vi "X_Overlay Dashed Line.vi"(4 "Dash Length (0)":u32, 6 "Color":u32, 7 "Overlay Group":string, 8 "error in (no error)":errorcluster, 9 "Point 2":T2, 10 "Point 1":T2, 11 "Refnum in":T1) -> (0 "error out":errorcluster, 3 "Refnum out":T1)   [LabVIEW 2021, in "Image.lvlib"]
uses:
  <vilib>/vision/Image Controls.llb/IMAQ Image.ctl
  Image.lvlib
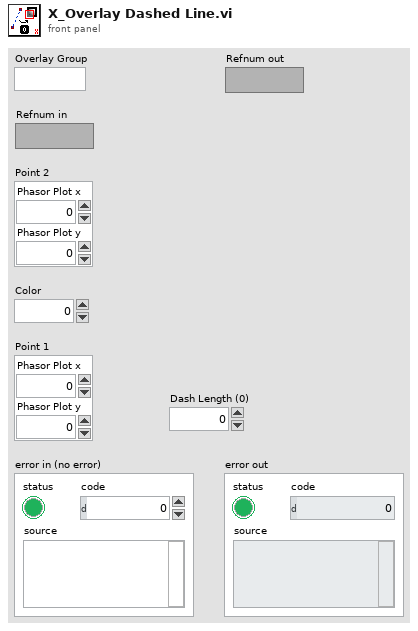
[diagram p1: front panel]
types:
  T1 = typedef "IMAQ Image.ctl" = refnum<image>
  T2 = cluster{"Phasor Plot x":i32, "Phasor Plot y":i32}
  T3 = cluster{"Phasor Plot x":i32, "Phasor Plot y":i32}[]
  T4 = cluster{"Phasor Plot x":dbl, "Phasor Plot y":dbl}
  T5 = cluster{"Phasor Plot x":dbl, "Phasor Plot y":dbl}[]
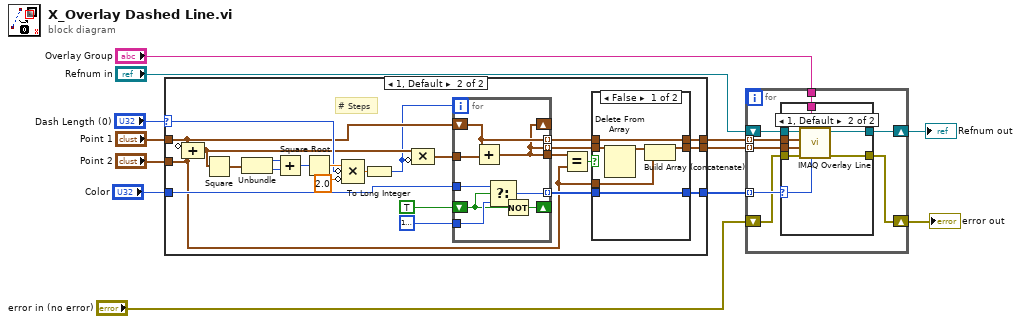
[diagram p0: block diagram]
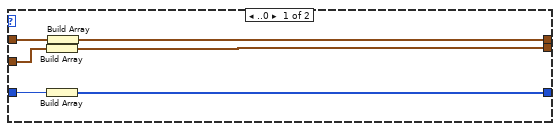
[diagram p2: hidden frame]
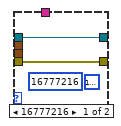
[diagram p4: hidden frame]
diagram:
  n1 = case shown="1, Default" "Dash Length (0)" {
    selector: "Dash Length (0)" -> [_ w37]
    tunnel: "Point 1" -> [w18 w35]
    tunnel: "Point 2" -> [w16 w19]
    tunnel: [w17 w23] -> w4
    tunnel: [w15 w22] -> w3
    tunnel: "Color" -> [w14 w33]
    tunnel: [w13 w20] -> w1
    frame ..0 {
      n2 = Build Array(w16) -> (w15:T3)
      n3 = Build Array(w14) -> (w13:u32[])
      n4 = Build Array(w18) -> (w17:T3)
    }
    frame 1, Default {
      # "# Steps"
      n5 = Compound Arithmetic op=ADD(invert w35, w19) -> (w30:T2)
      n6 = Square(x=w30) -> (x^2=w42:T2)
      n7 = Unbundle(w42) -> ("Phasor Plot x"=w41:i32, "Phasor Plot y"=w40:i32)
      n8 = Add(x=w41, y=w40) -> (x+y=w39:i32)
      n9 = Square Root(x=w39) -> (sqrt(x)=w38:dbl)
      n10 = Compound Arithmetic op=MULTIPLY(w38, invert w37, invert 2.0 ("value")) -> (w31:dbl)
      n11 = To Long Integer(number=w31) -> (32bit integer=w29:i32)
      n12 = Compound Arithmetic op=MULTIPLY(w30, invert w29) -> (w28:T4)
      n13 = for {
        N: w29 -> [_]
        shift-right: [w52] -> _
        shift-left: w35 -> [w53]
        tunnel: [w53] -> w25 mode=indexing
        shift-right: [w55] -> _
        shift-left: TRUE -> [w56]
        tunnel: w33 -> [w59]
        tunnel: u32 16777216 -> [w58]
        tunnel: [w57] -> w21 mode=indexing
        tunnel: w28 -> [w54]
        tunnel: [w52] -> w24 mode=indexing
        tunnel: [w52] -> w27
        n14 = Add(x=w53, y=w54) -> (x+y=w52:T4)
        n15 = Select(t=w59, s=w56, f=w58) -> (s? t:f=w57:u32)
        n16 = Not(x=w56) -> (.not. x?=w55:bool)
      }
      n17 = Equal?(x=w27, y=w19) -> (x = y?=w26:bool)
      n18 = case shown="False" w26 {
        tunnel: w25 -> [w48 w51]
        tunnel: w24 -> [w46 w50]
        tunnel: [w48 w51] -> w23
        tunnel: [w44 w50] -> w22
        tunnel: w21 -> [w47 w49]
        tunnel: [w47 w49] -> w20
        tunnel: w19 -> [w43 _]
        frame False {
          n19 = Delete From Array(array=w46) -> (array with subset deleted=w45:T5)  [unwired: 2 in, 1 out]
          n20 = Build Array (concatenate)(w45, w43) -> (w44:T5)
        }
        frame True {
        }
      }
    }
  }
  n21 = for {
    tunnel: w1 -> [w67] mode=indexing
    tunnel: w3 -> [w66] mode=indexing
    tunnel: w4 -> [w65] mode=indexing
    tunnel: "Overlay Group" -> [w61]
    shift-right: [w63] -> w11
    shift-left: "error in (no error)" -> [w62]
    shift-right: [w64] -> w12
    shift-left: "Refnum in" -> [w60]
    n22 = case shown="1, Default" w67 {
      selector: w67 -> [_ w77]
      tunnel: w66 -> [_ w76]
      tunnel: w65 -> [_ w75]
      tunnel: [w69 w74] -> w64
      tunnel: [w68 w73] -> w63
      tunnel: w62 -> [w68 w72]
      tunnel: w61 -> [_ w71]
      tunnel: w60 -> [w69 w70]
      frame 16777216 {
        (unwired) u32 16777216
        (unwired) u32 16777216
      }
      frame 1, Default {
        n23 = call "IMAQ Overlay Line"("Color"=w77, "Group"=w71, "error in (no error)"=w72, "End Point"=w76, "Start Point"=w75, "Image"=w70) -> ("error out"=w73:errorcluster, "Image Out"=w74:T1)  [unwired: 4 in]
      }
    }
  }
  "Refnum out" <- w12
  "error out" <- w11
